vi "FaceEncodingsToArray.vi"(8 "error in (no error)":errorcluster, 11 "FaceEncodings in":refnum<k24>) -> (0 "error out":errorcluster, 2 "FaceEncodingArray":refnum<k24>[](array[refnum]), 3 "FaceEncodings out":refnum<k24>)   [LabVIEW 2020, in "FaceRecognitionDotNet.lvlib" / "FaceRecognition.lvclass"]
uses:
  FaceRecognition.lvclass
  dll/FaceRecognitionDotNet.dll
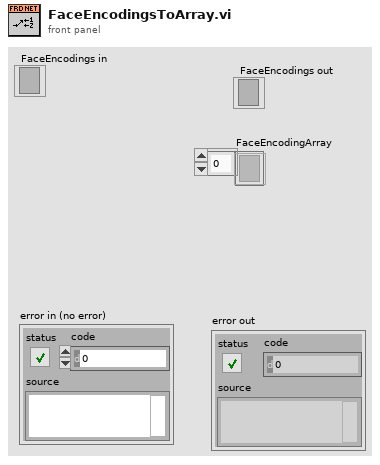
[diagram p1: front panel]
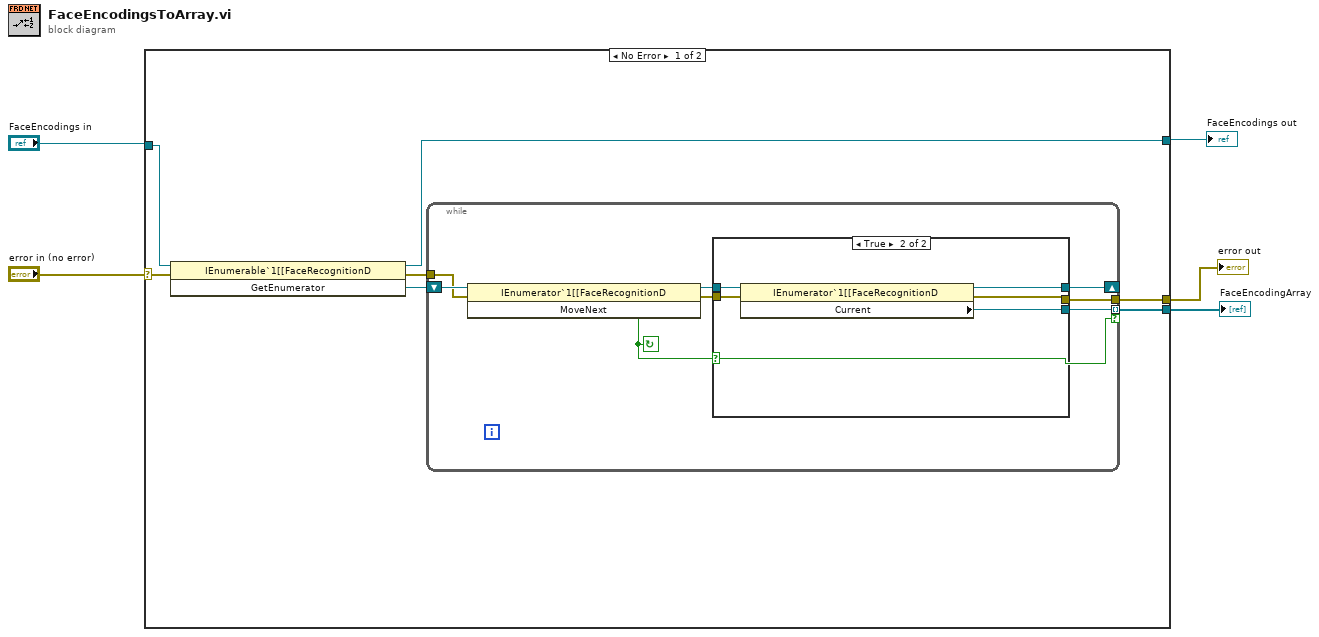
[diagram p0: block diagram]
diagram:
  n1 = case shown="No Error" "error in (no error)" {
    selector: "error in (no error)" -> [w8 w28]
    tunnel: "FaceEncodings in" -> [w6 w29]
    tunnel: [w12 w29] -> w5
    tunnel: [w9 w28] -> w4
    tunnel: [w7 _] -> w2
    frame No Error {
      n2 = invoke class="IEnumerable`1[[FaceRecognitionD" method="GetEnumerator"(reference=w6, error in=w8) -> (reference out=w12:refnum<k24>, error out=w11:errorcluster, "GetEnumerator"=w10:refnum<k24>)  [unwired: 1 in]
      n3 = while {
        tunnel: w11 -> [w18]
        shift-right: [w17] -> _
        shift-left: w10 -> [w20]
        tunnel: [w15] -> w9
        tunnel: [w13] -> w7 mode=indexing if=w14
        stop <- w14 continue-if-true
        n4 = invoke class="IEnumerator`1[[FaceRecognitionD" method="MoveNext"(reference=w20, error in=w18) -> (reference out=w19:refnum<k24>, error out=w16:errorcluster, "MoveNext"=w14:bool)  [unwired: 1 in]
        n5 = case shown="True" w14 {
          tunnel: w19 -> [w22 w27]
          tunnel: w16 -> [w21 w26]
          tunnel: [w22 w25] -> w17
          tunnel: [w21 w24] -> w15
          tunnel: [_ w23] -> w13
          frame False {
          }
          frame True {
            n6 = property class="IEnumerator`1[[FaceRecognitionD"(reference=w27, error in=w26) -> (reference out=w25:refnum<k24>, error out=w24:errorcluster, "Current"=w23:refnum<k24>)
          }
        }
      }
    }
    frame Error {
    }
  }
  "FaceEncodings out" <- w5
  "error out" <- w4
  "FaceEncodingArray" <- w2
